vi "Module Init.vi"(8 "error in (no error)":errorcluster, 11 "System Health Module in":refnum<class "System Health Module.lvclass">) -> (0 "error out":errorcluster, 3 "System Health Module out":refnum<class "System Health Module.lvclass">)   [LabVIEW 2020, in "Volatus.lvlib" / "System Health Module.lvclass"]
uses:
  System Health Module.lvclass
  System Health Module.lvclass/System Health Module.ctl
  Module/Module.lvclass
  C:/dev/lv20CE/relink/lv-volatus/Volatus/Module/Module.lvclass
  C:/dev/lv20CE/relink/lv-volatus/Volatus/System Health Module/System Health Module.lvclass
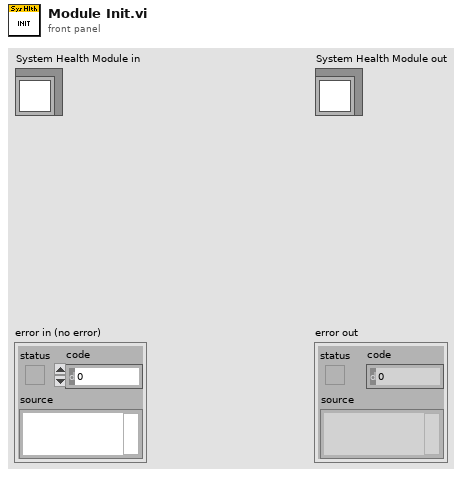
[diagram p1: front panel]
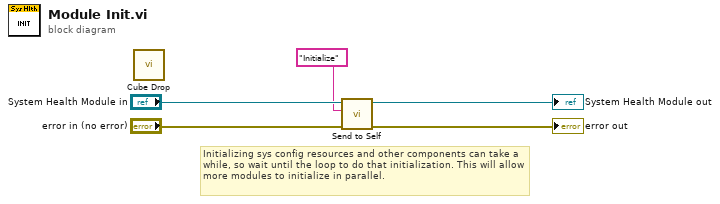
[diagram p0: block diagram]
diagram:
  # "Initializing sys config resources and other components can take a while, so wait until the loop to do that initialization. This will allow more modules to initialize in parallel."
  n1 = call "Cube Drop.vi"() -> ()  [unwired: 12 in]
  n2 = call "Send to Self.vi"("error in (no error)"="error in (no error)", "Message ID"="Initialize", "Module in"="System Health Module in") -> ("error out"=→"error out":errorcluster, "Module out"=→"System Health Module out":refnum<class "System Health Module.lvclass">)  [unwired: 7 in]
